vi "SDCP TMC FGV.vi"(3 "error in (no error)":errorcluster, 4 "RD/nWR":bool, 5 "TMC in":T1) -> (0 "error out":errorcluster, 2 "TMC out":T1)   [LabVIEW 2020]
uses:
  Typedefs/SDCP TMC Param.ctl
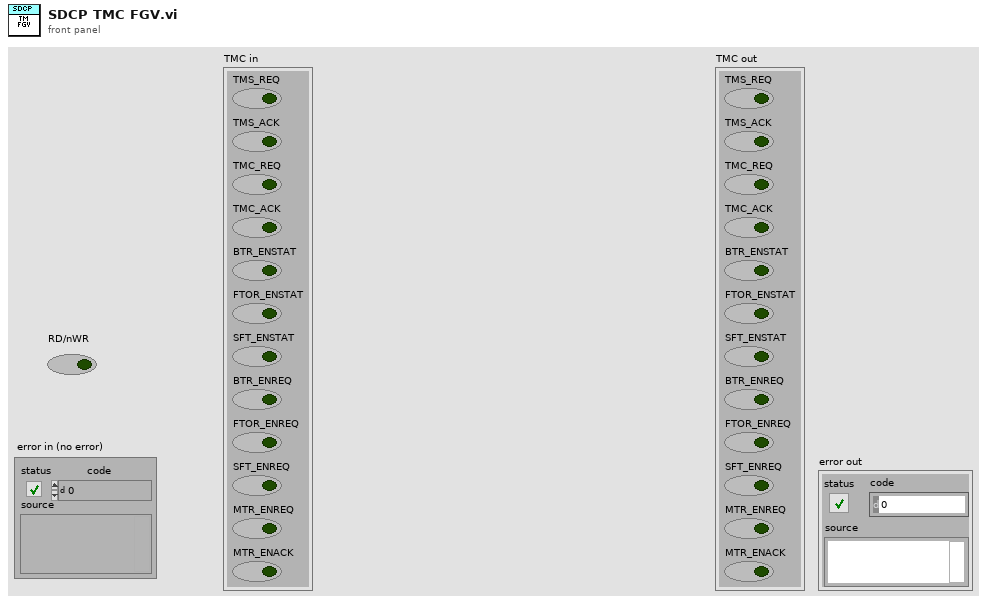
[diagram p1: front panel]
types:
  T1 = typedef "SDCP TMC Param.ctl" = cluster{"TMS_REQ":bool, "TMS_ACK":bool, "TMC_REQ":bool, "TMC_ACK":bool, "BTR_ENSTAT":bool, "FTOR_ENSTAT":bool, "SFT_ENSTAT":bool, "BTR_ENREQ":bool, "FTOR_ENREQ":bool, "SFT_ENREQ":bool, "MTR_ENREQ":bool, "MTR_ENACK":bool}
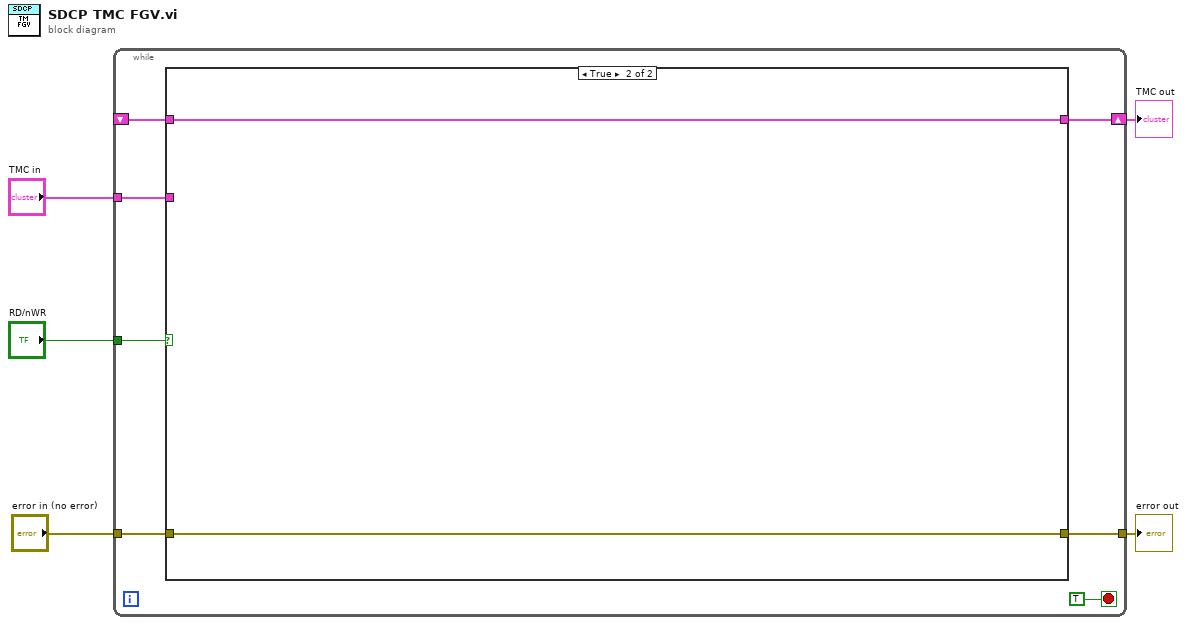
[diagram p0: block diagram]
diagram:
  n1 = while {
    tunnel: "error in (no error)" -> [w10]
    tunnel: "RD/nWR" -> [w11]
    shift-right: [w7] -> w2
    shift-left: _ -> [w6]
    tunnel: [w9] -> w1
    tunnel: "TMC in" -> [w8]
    stop <- TRUE stop-if-true
    n2 = case shown="True" w11 {
      tunnel: w10 -> [w14 w16]
      tunnel: [w14 w16] -> w9
      tunnel: w8 -> [w13 _]
      tunnel: [w13 w15] -> w7
      tunnel: w6 -> [_ w15]
      frame False {
      }
      frame True {
      }
    }
  }
  "TMC out" <- w2
  "error out" <- w1
